vi "_FPGA_DDS_BMem_of_Sine.vi"(9 "Cycle in":u16) -> (2 "sine":fxp<+,14,14>)   [LabVIEW 2018]
panel:
  out "Cross zero":bool
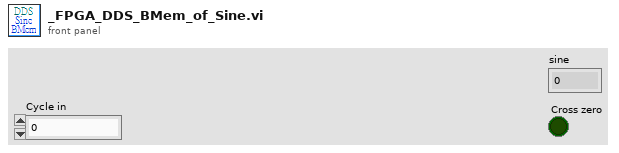
[diagram p1: front panel]
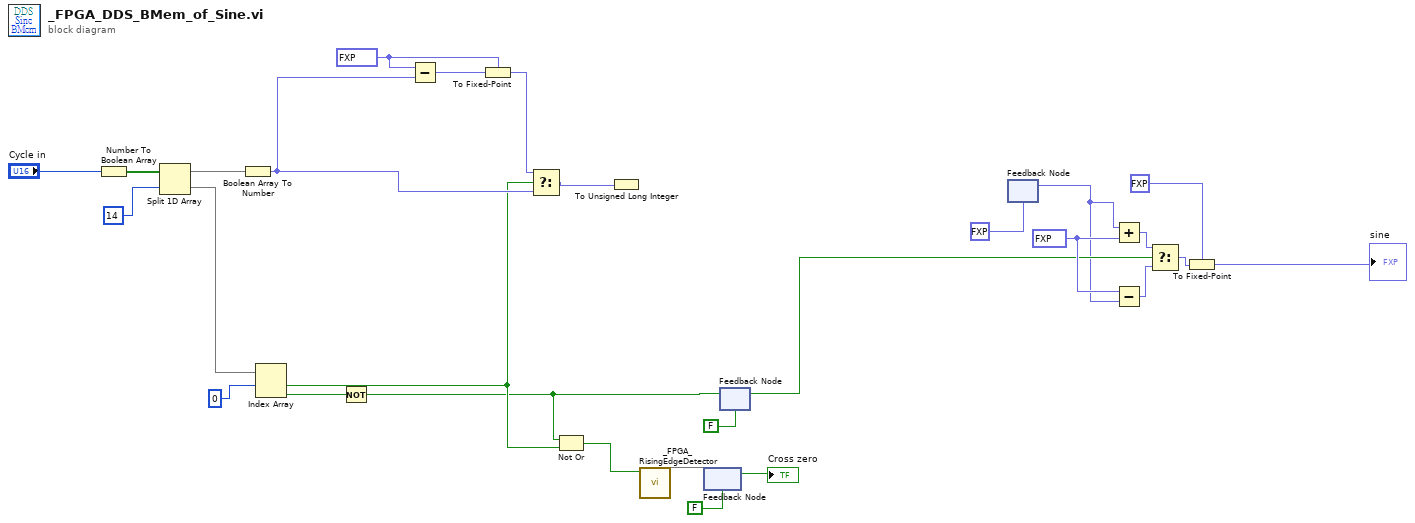
[diagram p0: block diagram]
diagram:
  w18 = fxp<+,14,14> 16383.0
  w19 = fxp<+,14,14> 8192.0
  n1 = Number To Boolean Array(number="Cycle in") -> (Boolean array=w28:bool[])
  n2 = Split 1D Array(array=w28, index=14) -> (first subarray=w26:bool[], second subarray=w21:bool[])
  n3 = Boolean Array To Number(Boolean array=w26) -> (number=w14:fxp<+,14,14>)
  n4 = Index Array(array=w21, index #1=0 ("index")) -> (element #1=w8:bool, element #2=w20:bool)  [unwired: 1 in]
  n5 = Not(x=w20) -> (.not. x?=w5:bool)
  n6 = Subtract(x=w18, y=w14) -> (x-y=w17:fxp<+/-,15,15>)
  n7 = To Fixed-Point(fixed-point type=w18, number=w17) -> (fixed-point=w16:fxp<+,14,14>)
  n8 = Select(t=w16, s=w8, f=w14) -> (s? t:f=w15:fxp<+,14,14>)
  n9 = Not Or(1:w8, 2:w5) -> (0:w7:bool)
  n10 = To Unsigned Long Integer(number=w15) -> ()  [unwired: 1 out]
  n11 = call "_FPGA_RisingEdgeDetector.vi"(11:w7) -> (3:w11)  [unwired: 9 in, 1 out]
  n12 = feedback-in #1(w11) -> ()
  n13 = feedback #1(FALSE ("Rising edge?")) -> (→"Cross zero":bool)
  n14 = feedback #2(FALSE ("Rising edge?")) -> (w4:bool)
  n15 = feedback-in #2(w5) -> ()
  n16 = feedback #3(fxp<+,14,14> 0.0 ("sine")) -> (w3:fxp<+,14,14>)
  n17 = feedback-in #3() -> (w1:fxp<+,14,14>)
  n18 = Add(x=w3, y=w19) -> (x+y=w23:fxp<+,15,15>)
  n19 = Subtract(x=w19, y=w3) -> (x-y=w22:fxp<+/-,15,15>)
  n20 = Select(t=w23, s=w4, f=w22) -> (s? t:f=w24:fxp<+/-,16,16>)
  n21 = To Fixed-Point(fixed-point type=fxp<+,14,14> 0.0 ("sine"), number=w24) -> (fixed-point=→"sine":fxp<+,14,14>)
